vi "RVC 3-link serial gantry.vi"() -> ()   [LabVIEW 2014]
uses:
  <vilib>/Analysis/Matrix/Datatypes/RealMatrix.ctl
  <vilib>/robotics/Kinematics/Analytical/Initialize Generic Serial Arm.vi
  <vilib>/robotics/Kinematics/Analytical/NI_Robotics_AnalyticKinematics.lvlib
  <vilib>/robotics/Kinematics/Robot/NI_Robotics_Serial Robot Arm.lvclass
  <vilib>/Analysis/Matrix/NI_Matrix.lvlib
panel:
  in  "appended array":dbl[](array[numeric])
  out "transformation":picture
  out "forward kinematics":T1
  out "3D Picture":refnum<vi>(3d-picture)
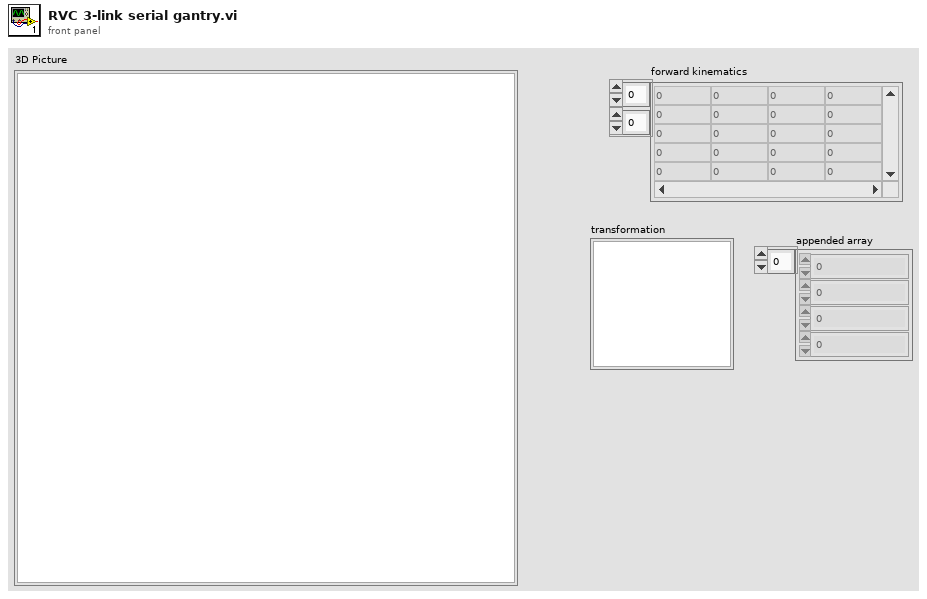
[diagram p1: front panel]
types:
  T1 = typedef "NI_Matrix.lvlib/RealMatrix.ctl" = dbl[][]
  T2 = typedef "DH Kinematic Parameters.ctl" = cluster{"twist angle":dbl, "length":dbl, "rotation angle":dbl, "offset distance":dbl, "joint type":T3, "joint coordinate offset":dbl}
  T3 = typedef "NI_Robotics_Link.lvclass/Joint Type.ctl" = enum16{"Revolute", "Prismatic"}
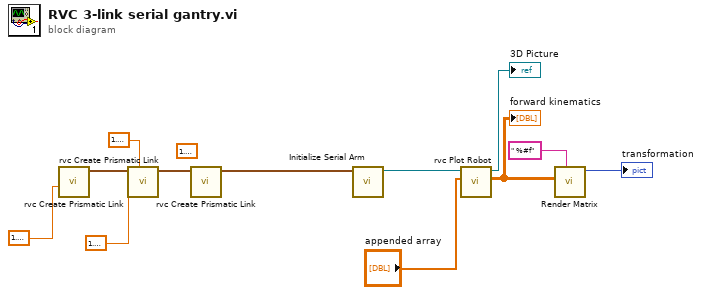
[diagram p0: block diagram]
diagram:
  (unwired) 1.5707963267948966
  n1 = call "rvc Create Prismatic Link.vi"("twist angle (alpha)"=1.5707963267948966) -> ("Array"=w4:T2[])  [unwired: 10 in]
  n2 = call "rvc Create Prismatic Link.vi"("rotation angle (theta)"=1.5707963267948966, "twist angle (alpha)"=1.5707963267948966, "Array 2"=w4) -> ("Array"=w6:T2[])  [unwired: 8 in]
  n3 = call "rvc Create Prismatic Link.vi"("Array 2"=w6) -> ("Array"=w5:T2[])  [unwired: 10 in]
  n4 = call-poly <vilib>:"Initialize Serial Arm.vi"("kinematic parameters"=w5) -> ("serial arm out"=w12:refnum<class "NI_Robotics_Serial Robot Arm.lvclass">)  [unwired: 9 in, 1 out]
  n5 = call "rvc Plot Robot.vi"("joint positions"="appended array", "NI_Robotics_Serial Robot Arm in"=w12) -> ("forward kinematics"=w8:T1, "Scene Object Out"=→"3D Picture":refnum<vi>)  [unwired: 7 in, 1 out]
  "forward kinematics" <- w8
  n6 = call "Render Matrix.vi"("format string"=" %#f", "A"=w8) -> ("picture out"=→"transformation":picture)  [unwired: 9 in]
